vi "Unconstrained Linear Fit.vi"(0 "Y":dbl[](array[numeric]) format="%#.6g", 5 "X":dbl[](array[numeric]) format="%#.6g", 7 "Weight":dbl[](array[numeric]) format="%#.6g", 9 "tolerance":dbl=0.0001, 11 "method":T1 items=["Least Square", "Least Absolute Residual", "Bisquare"]) -> (4 "Best Linear Fit":dbl[](array[numeric]) format="%#.6g", 6 "slope":dbl format="%#.6g", 8 "intercept":dbl format="%#.6g", 14 "residue":dbl format="%#.6g", 15 "error":i32)   [LabVIEW 2010, in "NI_AALPro.lvlib"]
doc: "Returns the linear fit of a data set (<B>X</B>, <B>Y</B>) using the Least Square, Least Absolute Residual, or Bisquare method."
uses:
  NI_AALPro.lvlib
  Curve Fitting Criteria.ctl
panel:
  # "Linear Fit"
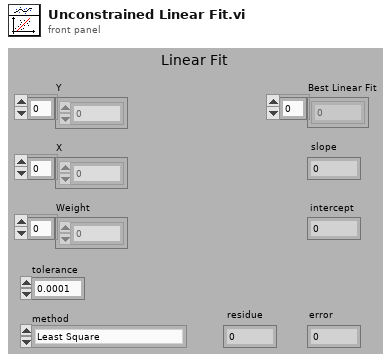
[diagram p1: front panel]
types:
  T1 = typedef "NI_AALPro.lvlib/Curve Fitting Criteria.ctl" = u16
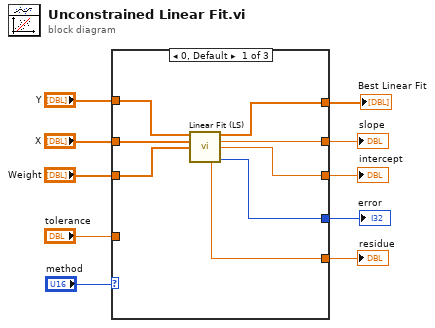
[diagram p0: block diagram]
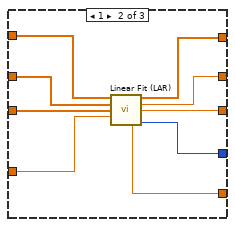
[diagram p2: hidden frame]
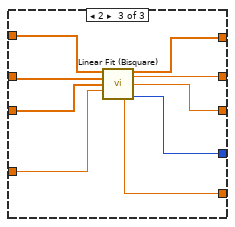
[diagram p3: hidden frame]
diagram:
  n1 = case shown="0, Default" "method" {
    tunnel: "Y" -> [w18 w27 w36]
    tunnel: "X" -> [w17 w26 w35]
    tunnel: [w14 w22 w31] -> w8
    tunnel: [w13 w21 w30] -> w7
    tunnel: [w12 w23 w29] -> w6
    tunnel: "Weight" -> [w16 w25 w34]
    tunnel: [w11 w20 w28] -> w4
    tunnel: [w15 w24 w32] -> w3
    tunnel: "tolerance" -> [_ w19 w33]
    frame 0, Default {
      n2 = call "Linear Fit (LS).vi"("Y"=w18, "X"=w17, "Weight"=w16) -> ("Best Linear Fit"=w15:dbl[], "slope"=w14:dbl, "intercept"=w13:dbl, "residue"=w11:dbl, "error"=w12:i32)  [unwired: 8 out]
    }
    frame 1 {
      n3 = call "Linear Fit (LAR).vi"("Y"=w27, "X"=w26, "Weight"=w25, "tol"=w19) -> ("Best Linear Fit"=w24:dbl[], "slope"=w22:dbl, "intercept"=w21:dbl, "residue"=w20:dbl, "error"=w23:i32)  [unwired: 7 out]
    }
    frame 2 {
      n4 = call "Linear Fit (Bisquare).vi"("Y"=w36, "X"=w35, "Weight"=w34, "tol"=w33) -> ("Best Linear Fit"=w32:dbl[], "slope"=w31:dbl, "intercept"=w30:dbl, "residue"=w28:dbl, "error"=w29:i32)  [unwired: 7 out]
    }
  }
  "slope" <- w8
  "intercept" <- w7
  "error" <- w6
  "residue" <- w4
  "Best Linear Fit" <- w3
